vi "Create Chans from typedefs.vi"(5 "Default from text? (F)":bool, 7 "Prevent overwrite? (F)":bool, 8 "error in":errorcluster, 9 "Type":T2, 10 "Ctl Ref":refnum<vi>, 11 "Section Ref in":T1 format="%.0x") -> (0 "error out":errorcluster, 2 "Section Refs":T1[](array[typedef]) format="%.0x", 3 "Section Ref out":T1 format="%.0x")   [LabVIEW 2016, in "DCM System Explorer.lvlib"]
uses:
  DCM System Explorer.lvlib
  <vilib>/NI Veristand/Custom Device API/Custom Device Item Ref.ctl
  <vilib>/NI Veristand/Custom Device API/Custom Device Channel Type.ctl
  Shared/DCM Constants and GUIDs.vi
  Custom Device Ref.vi
  <vilib>/NI VeriStand/Custom Device API/Custom Device API.lvlib
  DCM Shared.lvlib
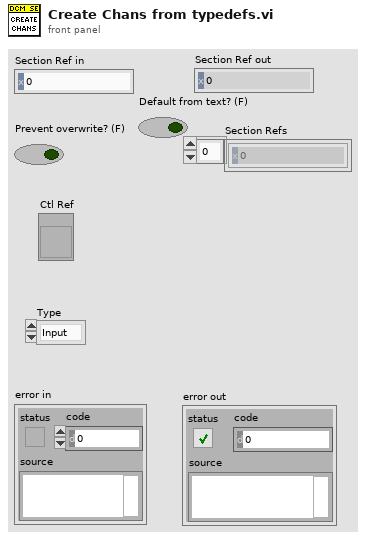
[diagram p1: front panel]
types:
  T1 = typedef "Custom Device API.lvlib/Custom Device Item Ref.ctl" = u64
  T2 = typedef "Custom Device API.lvlib/Custom Device Channel Type.ctl" = enum16{"Input", "Output"}
  T3 = cluster{"Ctl Ref":refnum<vi>, "Index Ref":refnum<vi>, "Array Refs":refnum<vi>[], "Array Positions":i32[][], "Device Ref":T1, "Section Ref":T1, "GUIDChDelProt":string, "GUIDSectDelProt":string}
  T4 = cluster{"Ctl Ref":refnum<vi>, "Index Ref":refnum<vi>, "Array Refs":refnum<vi>[], "Array Positions":i32[][], "Device Ref":T1, "Section Ref":T1, "GUIDChDelProt":string, "GUIDSectDelProt":string}[]
  T5 = typedef "Custom Device API.lvlib/Custom Device Channel.ctl" = cluster{"Type":T2, "Units":string, "Default Value":dbl, "Faultable":bool, "Scalable":bool}
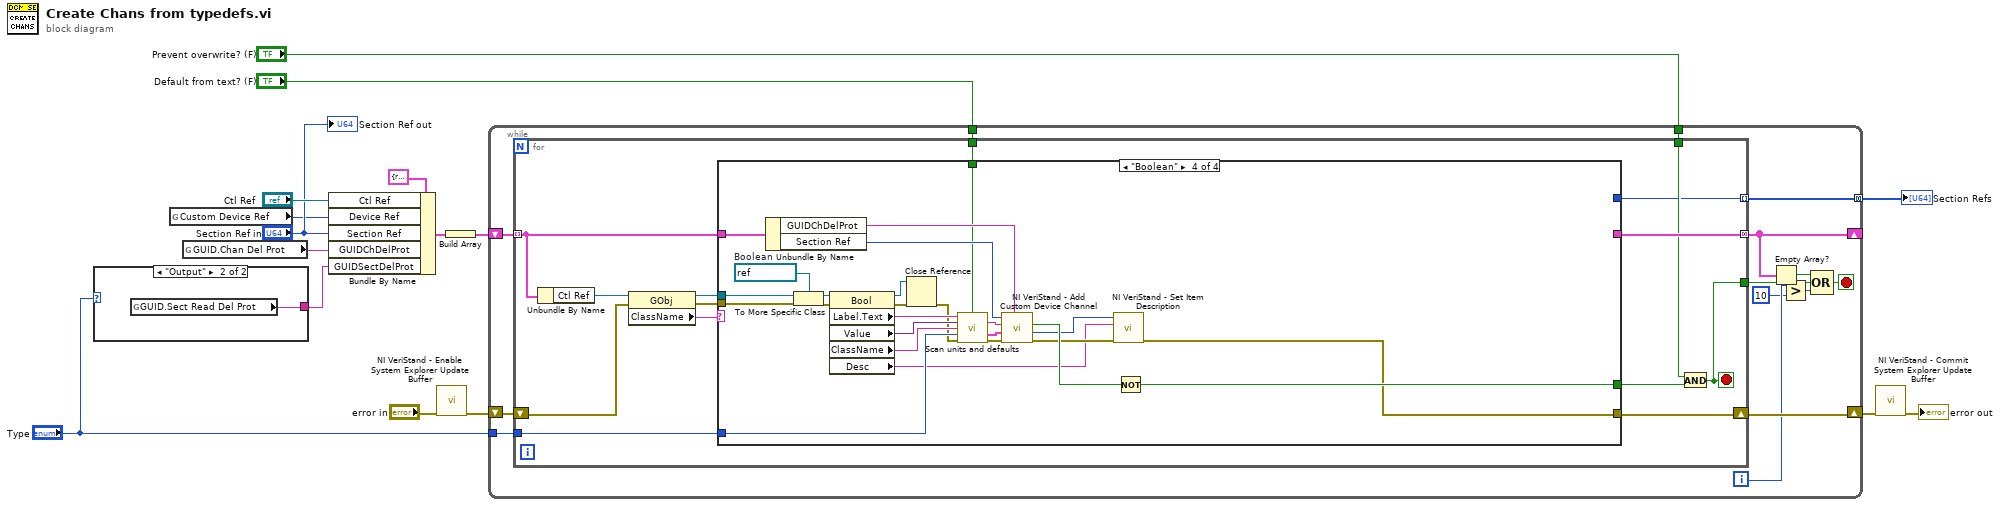
[diagram p0: block diagram]
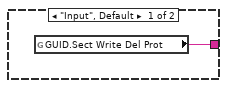
[diagram p2: hidden frame]
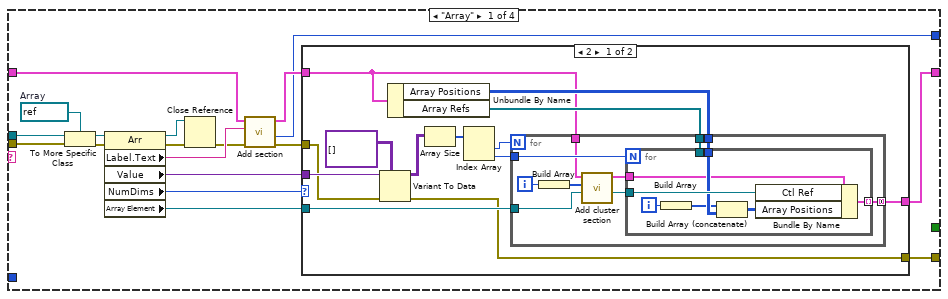
[diagram p3: hidden frame]
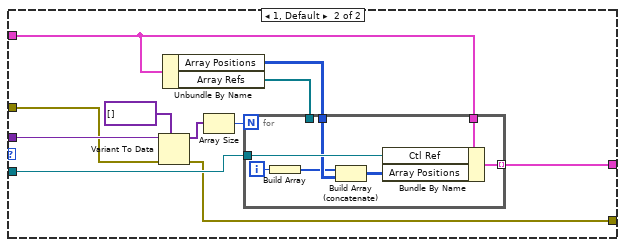
[diagram p4: hidden frame]
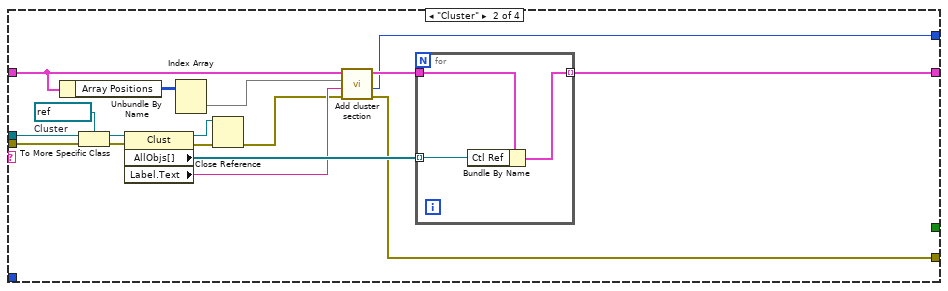
[diagram p5: hidden frame]
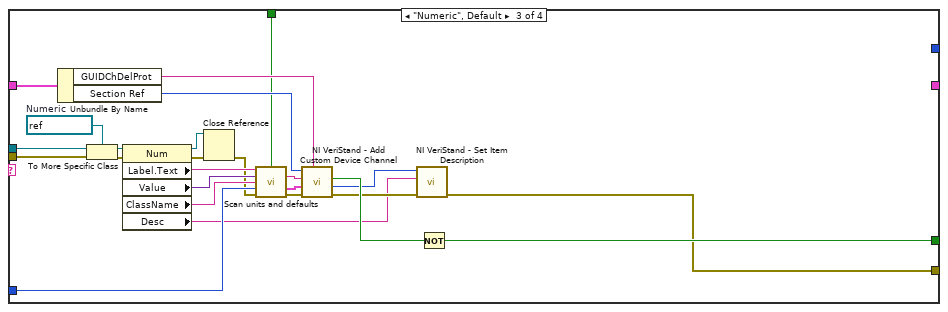
[diagram p6: hidden frame]
diagram:
  n1 = case shown="\"Output\"" "Type" {
    tunnel: [w17 w18] -> w8
    frame "Input", Default {
      n2 = global read "DCM Constants and GUIDs.vi" "GUID.Sect Write Del Prot"() -> (w17:string)
    }
    frame "Output" {
      n3 = global read "DCM Constants and GUIDs.vi" "GUID.Sect Read Del Prot"() -> (w18:string)
    }
  }
  n4 = global read "Custom Device Ref.vi" "Custom Device Ref"() -> (w5:T1)
  n5 = global read "DCM Constants and GUIDs.vi" "GUID.Chan Del Prot"() -> (w14:string)
  n6 = Bundle By Name(cluster=T3 {"Ctl Ref"=refnum, "Index Ref"=refnum, "Array Refs"=[], "Array Positions"=[], "Device Ref"=0, "Section Ref"=0, "GUIDChDelProt"="", "GUIDSectDelProt"=""} ("Data"), "Ctl Ref"="Ctl Ref", "Device Ref"=w5, "Section Ref"="Section Ref in", "GUIDChDelProt"=w14, "GUIDSectDelProt"=w8) -> (w15:T3)
  n7 = call <vilib>:"NI VeriStand - Enable System Explorer Update Buffer.vi"("error in (no error)"="error in") -> ("error out"=w3:errorcluster)  [unwired: 10 in]
  n8 = Build Array(w15) -> (w16:T4)
  n9 = while {
    shift-right: [w30] -> _
    shift-left: w16 -> [w32]
    tunnel: "Type" -> [w31]
    shift-right: [w29] -> w2
    shift-left: w3 -> [w28]
    tunnel: "Prevent overwrite? (F)" -> [w21]
    tunnel: "Default from text? (F)" -> [w20]
    tunnel: [w19] -> w9 mode=concatenating
    i -> [w24]
    stop <- w26 stop-if-true
    n10 = for {
      tunnel: w32 -> [w41] mode=indexing
      tunnel: w31 -> [w45]
      tunnel: [w44] -> w30 mode=concatenating
      shift-right: [w42] -> w29
      shift-left: w28 -> [w38]
      tunnel: [w37] -> w25
      tunnel: w21 -> [w35]
      tunnel: w20 -> [w34]
      tunnel: [w33] -> w19 mode=indexing
      stop <- w37 stop-if-true
      n11 = Unbundle By Name(w41) -> ("Ctl Ref"=w43:refnum<vi>)
      n12 = property class="GObj"(reference=w43, error in=w38) -> (reference out=w46:refnum<vi>, error out=w39:errorcluster, "ClassName"=w40:string)
      n13 = case shown="\"Numeric\", Default" w40 {
        tunnel: w46 -> [w64 w126 w156 w181]
        tunnel: w39 -> [w61 w125 w154 w179]
        tunnel: w45 -> [_ _ w141 w166]
        tunnel: [w56 w120 w132 w157] -> w42
        tunnel: w41 -> [w52 w119 w153 w178]
        tunnel: [w57 w123 _ _] -> w44
        tunnel: [_ _ w144 w169] -> w36
        tunnel: w34 -> [_ _ w139 w164]
        tunnel: [w50 w116 _ _] -> w33
        frame "Array" {
          w60 = refnum<vi> refnum  # Array
          n14 = To More Specific Class(target class=w60, reference=w64, error in=w61) -> (specific class reference=w63:refnum<vi>, error out=w62:errorcluster)
          n15 = property class="Arr"(reference=w63, error in=w62) -> (reference out=w49:refnum<vi>, error out=w48:errorcluster, "Label.Text"=w53:string, "Value"=w59:variant, "NumDims"=w58:u32, "Array Element"=w55:refnum<vi>)
          n16 = Close Reference(reference=w49, error in (no error)=w48) -> (error out=w47:errorcluster)
          n17 = call "Add section.vi"("error in"=w47, "Label.Text in"=w53, "Data in"=w52) -> ("error out"=w54:errorcluster, "Section Ptr"=w50:T1, "Data out"=w51:T3)  [unwired: 5 in, 1 out]
          n18 = case shown="2" w58 {
            tunnel: w59 -> [w75 w102]
            tunnel: w54 -> [w66 w94]
            tunnel: w51 -> [w65 w95]
            tunnel: [w71 w100] -> w57
            tunnel: [w69 w98] -> w56
            tunnel: w55 -> [w70 w99]
            frame 2 {
              n19 = Variant To Data(error in=w66, type=variant[][] [], Variant=w75) -> (data=w76:variant[][], error out=w69:errorcluster)
              n20 = Unbundle By Name(w65) -> ("Array Positions"=w68:i32[][], "Array Refs"=w67:refnum<vi>[])
              n21 = Array Size(array=w76) -> (size(s)=w74:i32[])
              n22 = Index Array(array=w74) -> (element #1=w73:i32, element #2=w72:i32)  [unwired: 2 in]
              n23 = for {
                N: w73 -> [_]
                tunnel: w72 -> [w86]
                tunnel: [w84] -> w71 mode=concatenating
                tunnel: w70 -> [w85]
                tunnel: w68 -> [w83]
                tunnel: w67 -> [w82]
                tunnel: w65 -> [w79]
                i -> [w81]
                n24 = Build Array(w81) -> (w78:i32[])
                n25 = call "Add cluster section.vi"("Array Positions (none)"=w78, "Data in"=w79) -> ("Data out"=w80:T3)  [unwired: 6 in, 3 out]
                n26 = for {
                  N: w86 -> [_]
                  tunnel: w85 -> [w91]
                  tunnel: [w92] -> w84 mode=indexing
                  tunnel: w83 -> [w89]
                  tunnel: w82 -> [_]
                  tunnel: w80 -> [w87]
                  i -> [w93]
                  n27 = Build Array(w93) -> (w88:i32[])
                  n28 = Build Array (concatenate)(w88, w89) -> (w90:i32[][])
                  n29 = Bundle By Name(cluster=w87, "Ctl Ref"=w91, "Array Positions"=w90) -> (w92:T3)
                }
              }
            }
            frame 1, Default {
              n30 = Variant To Data(error in=w94, type=variant[] [], Variant=w102) -> (data=w103:variant[], error out=w98:errorcluster)
              n31 = Unbundle By Name(w95) -> ("Array Positions"=w97:i32[][], "Array Refs"=w96:refnum<vi>[])
              n32 = Array Size(array=w103) -> (size(s)=w101:i32)
              n33 = for {
                N: w101 -> [_]
                tunnel: w95 -> [w111]
                tunnel: [w110] -> w100 mode=indexing
                tunnel: w99 -> [w108]
                tunnel: w97 -> [w106]
                tunnel: w96 -> [_]
                i -> [w109]
                n34 = Build Array(w109) -> (w105:i32[])
                n35 = Build Array (concatenate)(w105, w106) -> (w107:i32[][])
                n36 = Bundle By Name(cluster=w111, "Ctl Ref"=w108, "Array Positions"=w107) -> (w110:T3)
              }
            }
          }
        }
        frame "Cluster" {
          w124 = refnum<vi> refnum  # Cluster
          n37 = Unbundle By Name(w119) -> ("Array Positions"=w118:i32[][])
          n38 = To More Specific Class(target class=w124, reference=w126, error in=w125) -> (specific class reference=w128:refnum<vi>, error out=w127:errorcluster)
          n39 = property class="Clust"(reference=w128, error in=w127) -> (reference out=w114:refnum<vi>, error out=w113:errorcluster, "AllObjs[]"=w121:refnum<vi>[], "Label.Text"=w115:string)
          n40 = Index Array(array=w118) -> (element=w117:i32[])  [unwired: 2 in]
          n41 = Close Reference(reference=w114, error in (no error)=w113) -> (error out=w112:errorcluster)
          n42 = call "Add cluster section.vi"("error in (no error)"=w112, "Name (none)"=w115, "Array Positions (none)"=w117, "Data in"=w119) -> ("error out"=w120:errorcluster, "Section Ptr"=w116:T1, "Data out"=w122:T3)  [unwired: 4 in, 1 out]
          n43 = for {
            tunnel: w122 -> [w130]
            tunnel: w121 -> [w129] mode=indexing
            tunnel: [w131] -> w123 mode=indexing
            n44 = Bundle By Name(cluster=w130, "Ctl Ref"=w129) -> (w131:T3)
          }
        }
        frame "Numeric", Default {
          w148 = refnum<vi> refnum  # Numeric
          n45 = Unbundle By Name(w153) -> ("GUIDChDelProt"=w150:string, "Section Ref"=w149:T1)
          n46 = To More Specific Class(target class=w148, reference=w156, error in=w154) -> (specific class reference=w155:refnum<vi>, error out=w147:errorcluster)
          n47 = property class="Num"(reference=w155, error in=w147) -> (reference out=w134:refnum<vi>, error out=w135:errorcluster, "Label.Text"=w143:string, "Value"=w142:variant, "ClassName"=w140:string, "Desc"=w136:string)
          n48 = Close Reference(reference=w134, error in (no error)=w135) -> (error out=w133:errorcluster)
          n49 = call "Scan units and defaults.vi"("Name [Units] (default value)"=w143, "Default from text? (F)"=w139, "Default"=w142, "Classname"=w140, "Type"=w141, "error in"=w133) -> ("Name out"=w145:string, "Channel"=w152:T5, "error out"=w151:errorcluster)  [unwired: 7 in]
          n50 = call <vilib>:"NI VeriStand - Add Custom Device Channel.vi"("GUID (Default Channel)"=w150, "error in (no error)"=w151, "Channel"=w152, "Channel Name"=w145, "Parent Ref in"=w149) -> ("error out"=w137:errorcluster, "Channel Ref"=w138:T1, "Newly Created?"=w146:bool)  [unwired: 3 in, 1 out]
          n51 = call <vilib>:"NI VeriStand - Set Item Description.vi"("error in (no error)"=w137, "Description"=w136, "Item Ref in"=w138) -> ("error out"=w132:errorcluster)  [unwired: 6 in, 2 out]
          n52 = Not(x=w146) -> (.not. x?=w144:bool)
        }
        frame "Boolean" {
          w173 = refnum<vi> refnum  # Boolean
          n53 = Unbundle By Name(w178) -> ("GUIDChDelProt"=w175:string, "Section Ref"=w174:T1)
          n54 = To More Specific Class(target class=w173, reference=w181, error in=w179) -> (specific class reference=w180:refnum<vi>, error out=w172:errorcluster)
          n55 = property class="Bool"(reference=w180, error in=w172) -> (reference out=w159:refnum<vi>, error out=w160:errorcluster, "Label.Text"=w168:string, "Value"=w167:variant, "ClassName"=w165:string, "Desc"=w161:string)
          n56 = Close Reference(reference=w159, error in (no error)=w160) -> (error out=w158:errorcluster)
          n57 = call "Scan units and defaults.vi"("Name [Units] (default value)"=w168, "Default from text? (F)"=w164, "Default"=w167, "Classname"=w165, "Type"=w166, "error in"=w158) -> ("Name out"=w170:string, "Channel"=w177:T5, "error out"=w176:errorcluster)  [unwired: 7 in]
          n58 = call <vilib>:"NI VeriStand - Add Custom Device Channel.vi"("GUID (Default Channel)"=w175, "error in (no error)"=w176, "Channel"=w177, "Channel Name"=w170, "Parent Ref in"=w174) -> ("error out"=w162:errorcluster, "Channel Ref"=w163:T1, "Newly Created?"=w171:bool)  [unwired: 3 in, 1 out]
          n59 = call <vilib>:"NI VeriStand - Set Item Description.vi"("error in (no error)"=w162, "Description"=w161, "Item Ref in"=w163) -> ("error out"=w157:errorcluster)  [unwired: 6 in, 2 out]
          n60 = Not(x=w171) -> (.not. x?=w169:bool)
        }
      }
      n61 = And(x=w35, y=w36) -> (x .and. y?=w37:bool)
    }
    n62 = Empty Array?(array=w30) -> (empty?=w27:bool)
    n63 = Greater?(x=w24, y=10) -> (0:w22:bool)
    n64 = Compound Arithmetic op=OR(w27, w25, w22) -> (w26:bool)
  }
  "Section Refs" <- w9
  n65 = call <vilib>:"NI VeriStand - Commit System Explorer Update Buffer.vi"("error in (no error)"=w2) -> ("error out"=→"error out":errorcluster)  [unwired: 10 in]
  "Section Ref out" <- "Section Ref in"
